vi "WLAN_FrameAnalysis - Optimized.vi"(8 "error in (no error)":errorcluster, 10 "Decode SC":bool, 11 "input cluster":cluster{"t0":dbl, "dt":dbl, "Y":cdb[]}) -> (0 "error out":errorcluster, 1 "Constellation":cdb[](graph), 2 "Modulation parameter":T1, 3 "output bits":i8[](array[numeric]), 4 "Frequency offset":dbl, 5 "SIG valid?":bool)   [LabVIEW 2022 SP3]
panel:
  out "x+y":dbl
  out "Frequency offset(LTF)":dbl
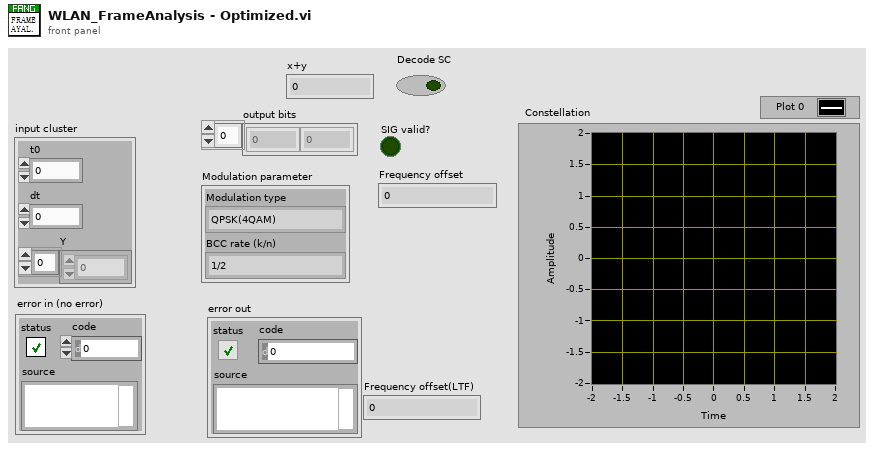
[diagram p1: front panel]
types:
  T1 = cluster{"Modulation type":enum16{"QPSK(4QAM)", "64QAM", "16QAM", "BPSK"}, "BCC rate (k/n)":enum16{"1/2", "2/3", "3/4"}}
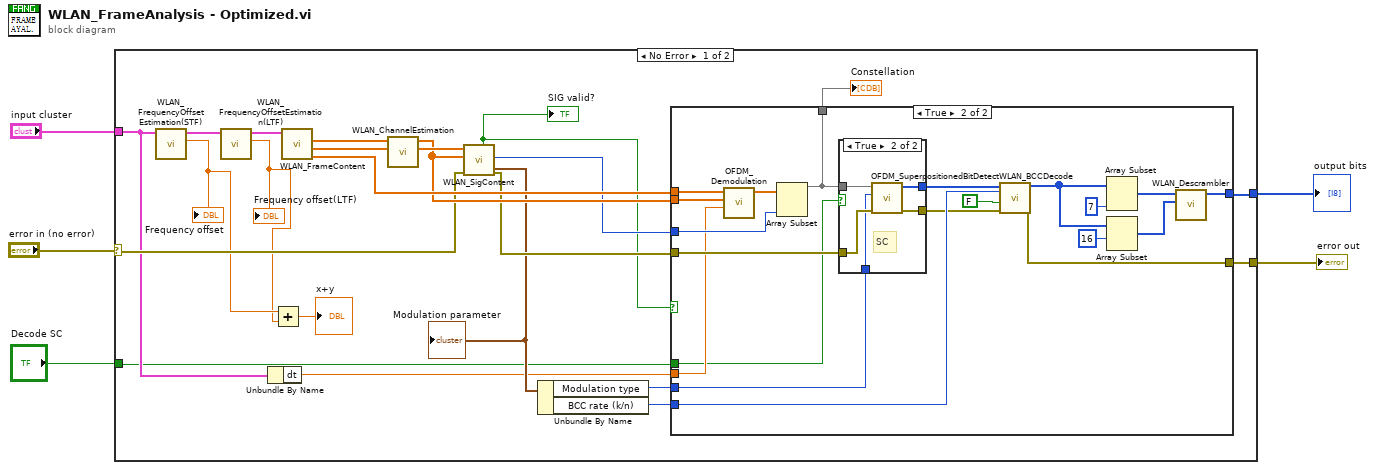
[diagram p0: block diagram]
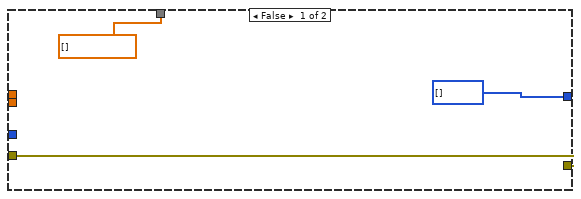
[diagram p2: hidden frame]
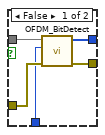
[diagram p3: hidden frame]
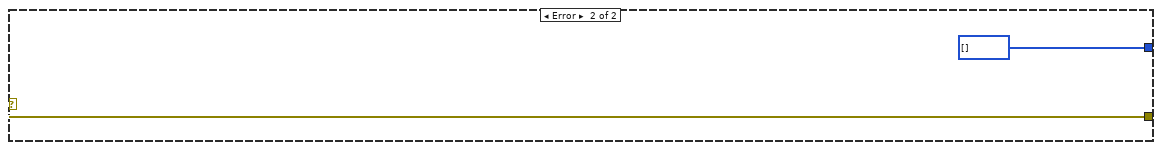
[diagram p4: hidden frame]
diagram:
  n1 = case shown="No Error" "error in (no error)" {
    selector: "error in (no error)" -> [w14 w61]
    tunnel: "input cluster" -> [w8 _]
    tunnel: [w21 w61] -> w4
    tunnel: [w20 i8[] [] ("scrambled bits")] -> w3
    tunnel: "Decode SC" -> [w6 _]
    frame No Error {
      n2 = call "WLAN_FrequencyOffsetEstimation(STF).vi"("output cluster"=w8) -> ("Frequency offset(STF)"=w12:dbl, "output cluster 2"=w13:cluster{"t0":dbl, "dt":dbl, "Y":cdb[]})  [unwired: 8 in]
      "Frequency offset" <- w12
      n3 = call "WLAN_FrequencyOffsetEstimation(LTF).vi"("input cluster"=w13) -> ("Frequency offset(LTF)"=w11:dbl, "output cluster"=w9:cluster{"t0":dbl, "dt":dbl, "Y":cdb[]})  [unwired: 9 in]
      "Frequency offset(LTF)" <- w11
      n4 = Unbundle By Name(w8) -> ("dt"=w7:dbl)
      n5 = Add(x=w12, y=w11) -> (x+y=→"x+y":dbl)
      n6 = call "WLAN_FrameContent.vi"("Input cluster"=w9) -> ("DATA"=w27:cdb[], "SIG"=w25:cdb[], "LTF"=w26:cdb[])  [unwired: 7 in, 1 out]
      n7 = call "WLAN_ChannelEstimation.vi"("LTF"=w26) -> ("Frequency estimation"=w24:cdb[])  [unwired: 10 in]
      n8 = call "WLAN_SigContent.vi"("error in (no error)"=w14, "Frequency channel estimation"=w24, "SIG"=w25) -> ("error out"=w23:errorcluster, "Symbol numbers"=w22:i32, "Modulation parameter"=w19:T1, "SIG valid?"=w15:bool)  [unwired: 3 in, 2 out]
      "Modulation parameter" <- w19
      "SIG valid?" <- w15
      n9 = Unbundle By Name(w19) -> ("Modulation type"=w18:enum16{"QPSK(4QAM)", "64QAM", "16QAM", "BPSK"}, "BCC rate (k/n)"=w17:enum16{"1/2", "2/3", "3/4"})
      n10 = case shown="True" w15 {
        tunnel: w27 -> [_ w50]
        tunnel: [w30 w42] -> w21
        tunnel: w24 -> [_ w48]
        tunnel: w23 -> [w30 w47]
        tunnel: w22 -> [_ w46]
        tunnel: w18 -> [_ w45]
        tunnel: [i8[] [] ("scrambled bits") w33] -> w20
        tunnel: w17 -> [_ w44]
        tunnel: [cdb[] [] w36] -> w16
        tunnel: w7 -> [_ w32]
        tunnel: w6 -> [_ w31]
        frame False {
        }
        frame True {
          n11 = call "OFDM_Demodulation.vi"("sampling period"=w32, "Frequency channel estimation"=w48, "Input sequence"=w50) -> ("Output sequence"=w49:cdb[])  [unwired: 7 in, 1 out]
          n12 = Array Subset(array=w49, length=w46) -> (w36:cdb[])  [unwired: 1 in]
          n13 = case shown="True" w31 {
            tunnel: w47 -> [w55 w58]
            tunnel: w45 -> [w54 w57]
            tunnel: [w53 w56] -> w43
            tunnel: w36 -> [w52 w59]
            tunnel: [w51 w60] -> w35
            frame False {
              n14 = call "OFDM_BitDetect.vi"("Input symbols"=w52, "Modulation type"=w54, "error in (no error)"=w55) -> ("Output bits"=w51:i8[], "error out"=w53:errorcluster)  [unwired: 6 in]
            }
            frame True {
              # "SC"
              n15 = call "OFDM_SuperpositionedBitDetect.vi"("Input symbols"=w59, "Modulation type"=w57, "error in (no error)"=w58) -> ("Output bits"=w60:i8[], "error out"=w56:errorcluster)  [unwired: 6 in]
            }
          }
          n16 = call "WLAN_BCCDecode.vi"("error in (no error)"=w43, "need add zeros?"=FALSE, "BCC rate (k/n)"=w44, "input bit stream"=w35) -> ("error out"=w42:errorcluster, "output bit stream"=w34:i8[])  [unwired: 6 in]
          n17 = Array Subset(array=w34, length=7) -> (w38:i8[])  [unwired: 1 in]
          n18 = Array Subset(array=w34, index=16) -> (w39:i8[])  [unwired: 1 in]
          n19 = call "WLAN_Descrambler.vi"("scrambler initial bits"=w38, "data bits"=w39) -> ("scrambled bits"=w33:i8[])  [unwired: 7 in]
        }
      }
      "Constellation" <- w16
    }
    frame Error {
    }
  }
  "error out" <- w4
  "output bits" <- w3
